vi "Set Attributes.vi"(4 "Private":bool[](array[boolean]), 5 "Update Pointer":bool[](array[boolean]), 6 "Pointer":bool[](array[boolean]), 7 "Unique ID":string, 8 "error in (no error)":errorcluster, 9 "Data":variant[](array[variant]), 10 "Name":string[](array[string]), 11 "Linked List in":refnum<class "Linked List.lvclass">) -> (0 "error out":errorcluster, 1 "Replaced?":bool[](array[boolean]), 2 "Unique IDs":string[](array[string]), 3 "Linked List out":refnum<class "Linked List.lvclass">)   [LabVIEW 2017, in "Linked Lists.lvlib" / "Linked List.lvclass"]
uses:
  <vilib>/gpm_packages/@cs/linked-list/Source/Linked List/Linked List/Linked List.lvclass
  <vilib>/gpm_packages/@cs/linked-list/Source/Linked List/Linked List Definition/Linked List Definition.lvclass
  <vilib>/gpm_packages/@cs/linked-list/Source/Linked List/Linked List/Linked List.lvclass/Linked List.ctl
  <vilib>/gpm_packages/@cs/lookup-table/Source/LookupTable/LookupTable.lvclass/LookupTable.ctl
  beab1386-fb03-4602-991d-c6dd99164584.vi
  9234b839-9e59-4810-9b93-2cc1a6eba5e0.vi
  59a1f23b-fdbe-4f7d-b72d-8891baf83f2c.vi
  <vilib>/gpm_packages/@cs/lookup-table/Source/LookupTable/Read Table Reference.vi
  beab1386-fb03-4602-991d-c6dd99164584.vi/966a8a0e-3ae3-4961-b435-a300f58fb250.vi
  9234b839-9e59-4810-9b93-2cc1a6eba5e0.vi/9ff51364-1b5e-4e05-a5c2-79c18ce53446.vi
  59a1f23b-fdbe-4f7d-b72d-8891baf83f2c.vi/01b992a5-4571-46d1-a751-44075d9d9044.vi
  <vilib>/gpm_packages/@cs/lookup-table/Source/LookupTable/LookupTable.lvclass
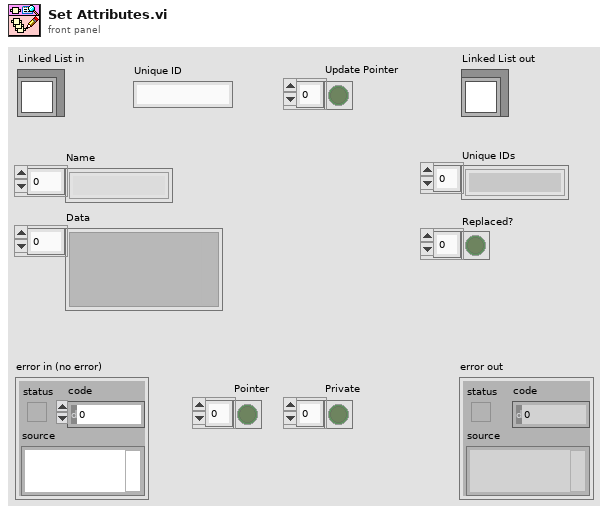
[diagram p1: front panel]
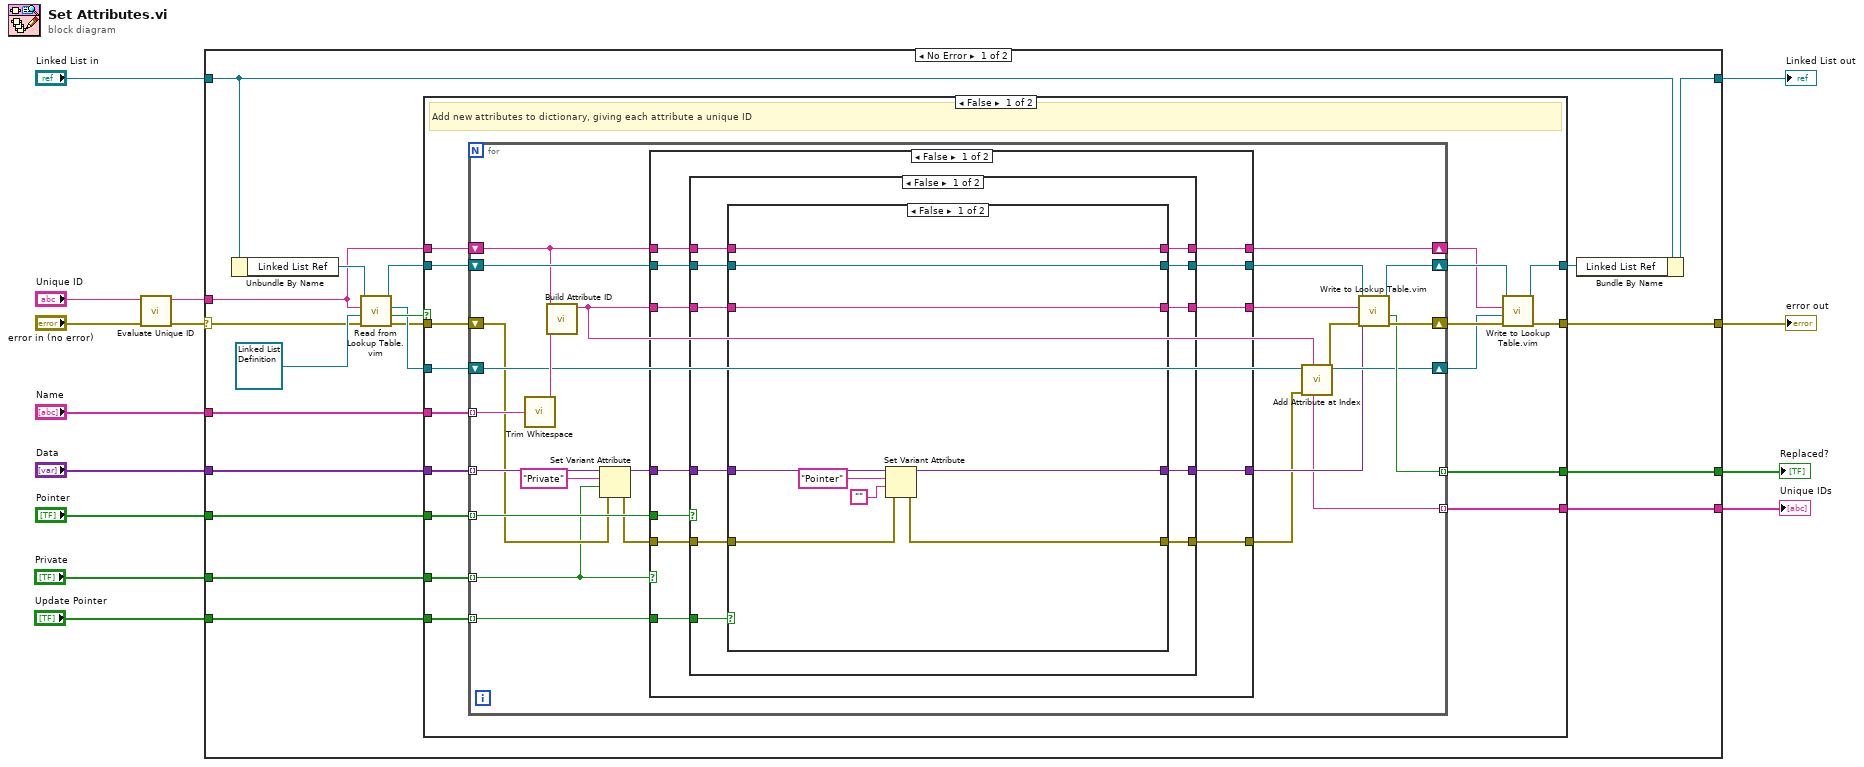
[diagram p0: block diagram]
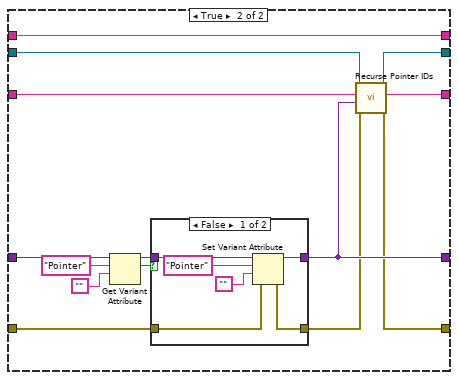
[diagram p2: hidden frame]
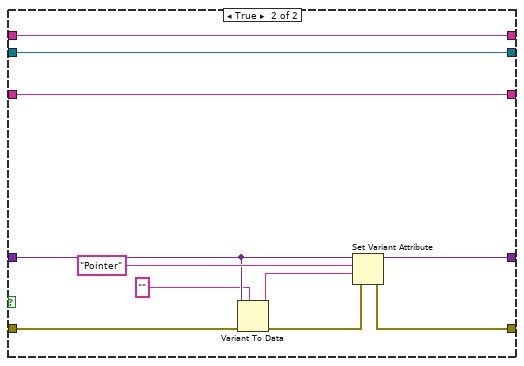
[diagram p4: hidden frame]
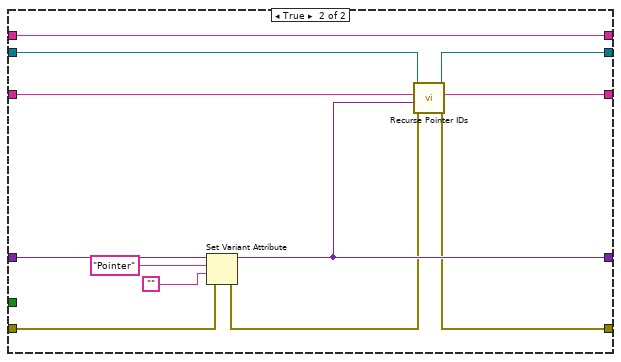
[diagram p5: hidden frame]
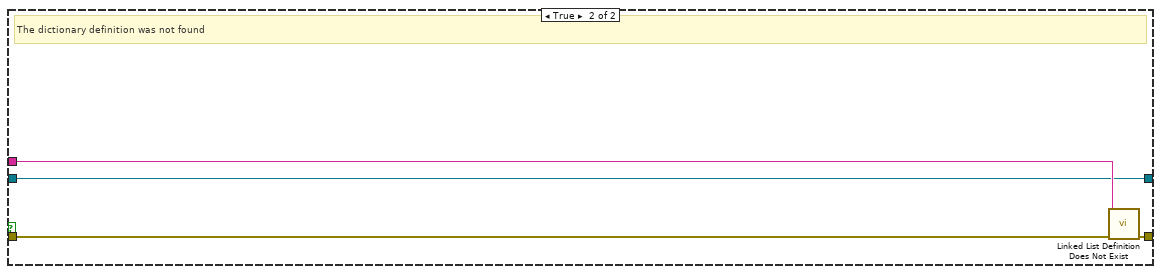
[diagram p6: hidden frame]
diagram:
  n1 = call <vilib>:"Evaluate Unique ID.vi"("error in (no error)"="error in (no error)", "Unique ID"="Unique ID") -> ("error out"=w11:errorcluster, "Unique ID Out"=w9:string)  [unwired: 8 in]
  n2 = case shown="No Error" w11 {
    selector: w11 -> [w24 w156]
    tunnel: [w25 w157] -> w12
    tunnel: "Linked List in" -> [w26 w157]
    tunnel: w9 -> [w23 _]
    tunnel: [w22 w156] -> w8
    tunnel: "Name" -> [w21 _]
    tunnel: "Data" -> [w20 _]
    tunnel: [w19 _] -> w5
    tunnel: [w18 _] -> w4
    tunnel: "Pointer" -> [w17 _]
    tunnel: "Private" -> [w16 _]
    tunnel: "Update Pointer" -> [w15 _]
    frame No Error {
      n3 = Unbundle By Name(w26) -> ("Linked List Ref"=w33:refnum<data-value>)
      n4 = call "Read from Lookup Table.vim"("error in (no error)"=w24, "Type"=refnum<class "Linked List Definition.lvclass"> refnum ("Linked List.lvlib:Linked List Definition.lvclass"), "Item Name"=w23, "LookupTable Reference"=w33) -> ("error out"=w28:errorcluster, "Not Found?"=w31:bool, "Value"=w29:refnum<class "Linked List Definition.lvclass">, "LookupTable Reference Out"=w30:refnum<data-value>)  [unwired: 4 in]
      n5 = case shown="False" w31 {
        tunnel: w30 -> [w49 w152]
        tunnel: w29 -> [w45 _]
        tunnel: [w41 w154] -> w22
        tunnel: w28 -> [w50 w155]
        tunnel: w23 -> [w48 w153]
        tunnel: [w39 w152] -> w27
        tunnel: w21 -> [w47 _]
        tunnel: w20 -> [w46 _]
        tunnel: [w44 _] -> w19
        tunnel: [w43 _] -> w18
        tunnel: w17 -> [w36 _]
        tunnel: w16 -> [w35 _]
        tunnel: w15 -> [w34 _]
        frame False {
          # "Add new attributes to dictionary, giving each attribute a unique ID"
          n6 = for {
            shift-right: [w74] -> w42
            shift-left: w50 -> [w54]
            shift-right: [w73] -> w40
            shift-left: w49 -> [w63]
            tunnel: w47 -> [w72] mode=indexing
            tunnel: w46 -> [w56] mode=indexing
            shift-right: [w68] -> w37
            shift-left: w45 -> [w69]
            shift-right: [w60] -> w38
            shift-left: w48 -> [w61]
            tunnel: [w70] -> w44 mode=indexing
            tunnel: [w58] -> w43 mode=indexing
            tunnel: w36 -> [w66] mode=indexing
            tunnel: w35 -> [w52] mode=indexing
            tunnel: w34 -> [w51] mode=indexing
            n7 = call <vilib>:"Trim Whitespace.vi"("string"=w72) -> ("trimmed string"=w71:string)  [unwired: 1 in]
            n8 = call <vilib>:"Build Attribute ID.vi"("Attr Name"=w71, "Unique ID"=w61) -> ("Attr ID Out"=w58:string)  [unwired: 9 in]
            n9 = Set Variant Attribute(Variant=w56, name="Private", value=w52, error in=w54) -> (Variant out=w55:variant, error out=w53:errorcluster)  [unwired: 1 out]
            n10 = case shown="False" w52 {
              tunnel: w55 -> [w76 w146]
              tunnel: w66 -> [w86 _]
              tunnel: w53 -> [w85 w144]
              tunnel: [w84 w145] -> w65
              tunnel: [w83 w149] -> w64
              tunnel: w63 -> [w82 w150]
              tunnel: [w81 w147] -> w62
              tunnel: w61 -> [w80 w151]
              tunnel: [w79 w151] -> w60
              tunnel: [w78 w143] -> w59
              tunnel: w58 -> [w77 w148]
              tunnel: w51 -> [w75 _]
              frame False {
                n11 = case shown="False" w86 {
                  tunnel: [w92 w139] -> w84
                  tunnel: w76 -> [w90 w137]
                  tunnel: w85 -> [w97 w134]
                  tunnel: [w91 w132] -> w78
                  tunnel: [w95 w130] -> w83
                  tunnel: w82 -> [w96 w130]
                  tunnel: [w93 w131] -> w81
                  tunnel: w77 -> [w94 w131]
                  tunnel: [w88 w129] -> w79
                  tunnel: w80 -> [w89 w129]
                  tunnel: w75 -> [w87 _]
                  frame False {
                    n12 = case shown="False" w87 {
                      tunnel: w97 -> [w102 w120]
                      tunnel: w96 -> [w99 w119]
                      tunnel: [w99 w118] -> w95
                      tunnel: w94 -> [w98 w117]
                      tunnel: [w98 w116] -> w93
                      tunnel: [w103 w115] -> w92
                      tunnel: [w101 w113] -> w91
                      tunnel: w90 -> [w104 w112]
                      tunnel: [w100 w107] -> w88
                      tunnel: w89 -> [w100 w107]
                      frame False {
                        n13 = Set Variant Attribute(Variant=w104, name="Pointer", value="", error in=w102) -> (Variant out=w103:variant, error out=w101:errorcluster)  [unwired: 1 out]
                      }
                      frame True {
                        n14 = Get Variant Attribute(Variant=w112, name="Pointer", default value (empty Variant)="") -> (duplicate Variant=w111:variant, found=w108:bool)  [unwired: 1 in, 2 out]
                        n15 = case shown="False" w108 {
                          tunnel: w120 -> [w125 w127]
                          tunnel: [w123 w128] -> w115
                          tunnel: [w122 w127] -> w114
                          tunnel: w111 -> [w121 w128]
                          frame False {
                            n16 = Set Variant Attribute(Variant=w121, name="Pointer", value="", error in=w125) -> (Variant out=w123:variant, error out=w122:errorcluster)  [unwired: 1 out]
                          }
                          frame True {
                          }
                        }
                        n17 = call <vilib>:"Recurse Pointer IDs.vi"("error in (no error)"=w114, "Type"=w115, "ID"=w117, "Linked List Ref"=w119) -> ("error out"=w113:errorcluster, "ID out"=w116:string, "Linked List Ref out"=w118:refnum<data-value>)  [unwired: 5 in]
                      }
                    }
                  }
                  frame True {
                    n18 = Variant To Data(error in=w134, type="", Variant=w137) -> (data=w135:string, error out=w133:errorcluster)
                    n19 = Set Variant Attribute(Variant=w137, name="Pointer", value=w135, error in=w133) -> (Variant out=w139:variant, error out=w132:errorcluster)  [unwired: 1 out]
                  }
                }
              }
              frame True {
                n20 = Set Variant Attribute(Variant=w146, name="Pointer", value="", error in=w144) -> (Variant out=w145:variant, error out=w140:errorcluster)  [unwired: 1 out]
                n21 = call <vilib>:"Recurse Pointer IDs.vi"("error in (no error)"=w140, "Type"=w145, "ID"=w148, "Linked List Ref"=w150) -> ("error out"=w143:errorcluster, "ID out"=w147:string, "Linked List Ref out"=w149:refnum<data-value>)  [unwired: 5 in]
              }
            }
            n22 = call <vilib>:"Add Attribute at Index.vi"("Unique ID"=w58, "error in (no error)"=w59, "Linked List Definition in"=w69) -> ("error out"=w67:errorcluster, "Linked List Definition out"=w68:refnum<class "Linked List Definition.lvclass">)  [unwired: 7 in]
            n23 = call "Write to Lookup Table.vim"("error in (no error)"=w67, "Item"=w65, "Item Name"=w62, "LookupTable Reference"=w64) -> ("error out"=w74:errorcluster, "Replaced?"=w70:bool, "LookupTable Reference Out"=w73:refnum<data-value>)  [unwired: 5 in]
          }
          n24 = call "Write to Lookup Table.vim"("error in (no error)"=w42, "Item"=w37, "Item Name"=w38, "LookupTable Reference"=w40) -> ("error out"=w41:errorcluster, "LookupTable Reference Out"=w39:refnum<data-value>)  [unwired: 5 in, 1 out]
        }
        frame True {
          # "The dictionary definition was not found"
          n25 = call <vilib>:"Linked List Definition Does Not Exist.vi"("Error In"=w155, "Unique ID"=w153) -> ("Error Out"=w154:errorcluster)  [unwired: 9 in]
        }
      }
      n26 = Bundle By Name(cluster=w26, "Linked List Ref"=w27) -> (w25:refnum<class "Linked List.lvclass">)
    }
    frame Error {
    }
  }
  "error out" <- w8
  "Linked List out" <- w12
  "Replaced?" <- w5
  "Unique IDs" <- w4
